vi "Get Wheel Parameter by Name.vi"(8 "error in (no error)":errorcluster, 10 "parameter name":string, 11 "wheel in":refnum<class "NI_Robotics_Mecanum Wheel.lvclass">) -> (0 "error out":errorcluster, 1 "found?":bool, 2 "parameter value":variant, 3 "wheel out":refnum<class "NI_Robotics_Mecanum Wheel.lvclass">)   [LabVIEW 2017, in "NI_Robotics_Mecanum Wheel.lvclass"]
uses:
  <vilib>/robotics/Steering/Mecanum Wheel/NI_Robotics_Mecanum Wheel.lvclass
  <vilib>/robotics/Steering/Mecanum Wheel/NI_Robotics_Mecanum Wheel.lvclass/NI_Robotics_Mecanum Wheel.ctl
  <vilib>/robotics/Steering/Wheel/NI_Robotics_Wheel.lvclass
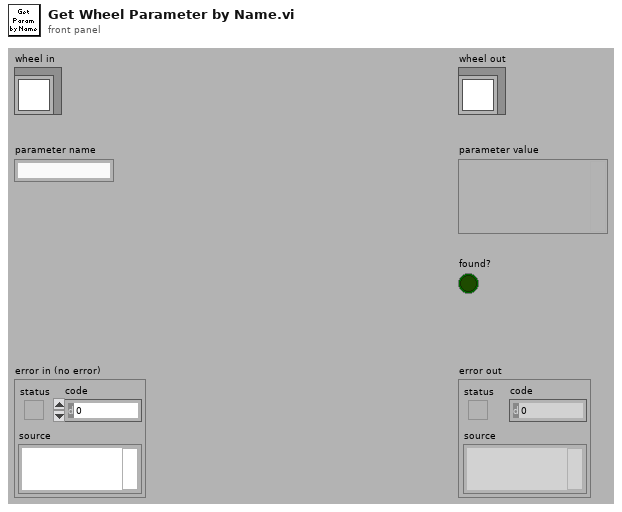
[diagram p1: front panel]
types:
  T1 = typedef "NI_Robotics_Mecanum Wheel.lvclass/Roller Orientation.ctl" = u16
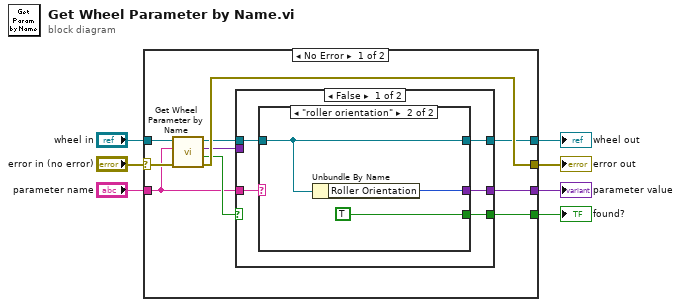
[diagram p0: block diagram]
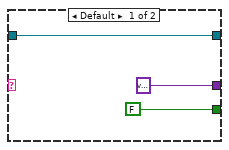
[diagram p2: hidden frame]
diagram:
  n1 = case shown="No Error" "error in (no error)" {
    selector: "error in (no error)" -> [w15 w32]
    tunnel: [w17 w32] -> w7
    tunnel: [w13 _] -> w6
    tunnel: [w11 _] -> w5
    tunnel: [w9 w33] -> w4
    tunnel: "parameter name" -> [w8 _]
    tunnel: "wheel in" -> [w16 w33]
    frame No Error {
      n2 = call-parent "Get Wheel Parameter by Name.vi"("error in (no error)"=w15, "parameter name"=w8, "wheel in"=w16) -> ("error out"=w17:errorcluster, "found?"=w14:bool, "parameter value"=w12:variant, "wheel out"=w10:refnum<class "NI_Robotics_Mecanum Wheel.lvclass">)  [unwired: 5 in]
      n3 = case shown="False" w14 {
        selector: w14 -> [_ w31]
        tunnel: [w19 w31] -> w13
        tunnel: w12 -> [_ w30]
        tunnel: [w18 w30] -> w11
        tunnel: w10 -> [w22 w29]
        tunnel: [w20 w29] -> w9
        tunnel: w8 -> [w21 _]
        frame False {
          n4 = case shown="\"roller orientation\"" w21 {
            tunnel: w22 -> [w25 w28]
            tunnel: [w25 w28] -> w20
            tunnel: [FALSE TRUE] -> w19
            tunnel: [variant ("parameter value") w27] -> w18
            frame Default {
            }
            frame "roller orientation" {
              n5 = Unbundle By Name(w28) -> ("Roller Orientation"=w27:T1)
            }
          }
        }
        frame True {
        }
      }
    }
    frame Error {
    }
  }
  "error out" <- w7
  "wheel out" <- w4
  "parameter value" <- w5
  "found?" <- w6
